vi "Configure.vi"(8 "error in (no error)":errorcluster, 9 "DAQ Parameters":T1={"Points Per A-Scan"=1024, "A-Scans Per B-Scan"=250, "Number of B-Scans"=1, "A-Scans Per Transfer"=1, "Trigger Voltage"=0.0, "Trigger Source"=enum."External", "Trigger Slope"=enum."Rising", "Channel"=enum."Channel 1", "Clock"=enum."Internal Clock", "Bits per Sample"=0.0, "Range"=0.0}, 10 "Scanning Parameters":T6={"Fast Axis Offset"=10.0, "Slow Axis Offset"=0.0, "Slow Axis Amp"=20.0, "Fast Axis Amp"=20.0, "Scan Pattern"=enum."Raster"} {"Fast Axis Amp" max=20 format="%#.2f"; "Slow Axis Amp" max=20 format="%#.2f"; "Slow Axis Offset" max=10 format="%#.2f"; "Fast Axis Offset" max=10 format="%#.2f"}, 11 "NI Galvo in":refnum<class "NI Galvo.lvclass">) -> (0 "error out":errorcluster, 3 "NI Galvo out":refnum<class "NI Galvo.lvclass">)   [LabVIEW 2014, in "NI Galvo.lvclass"]
uses:
  NI Galvo.lvclass
  Scanning Cluster.ctl
  DAQ/DAQ Parameters.ctl
  DAQ/Trigger Source.ctl
  DAQ/Trigger Slope.ctl
  Type Defs/OCT DAQ Channel Data Type.ctl
  DAQ/Clock Control.ctl
  Galvo.lvclass
  DAQ/DAQ Class.lvclass
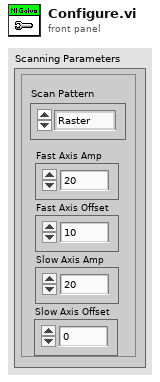
[diagram p1: front panel]
types:
  T1 = typedef "DAQ Class.lvclass/DAQ Parameters.ctl" = cluster{"Points Per A-Scan":u32, "A-Scans Per B-Scan":u32, "Number of B-Scans":u32, "A-Scans Per Transfer":u32, "Trigger Voltage":sgl, "Trigger Source":T2, "Trigger Slope":T3, "Channel":T4, "Clock":T5, "Bits per Sample":dbl, "Range":dbl}
  T2 = typedef "DAQ Class.lvclass/Trigger Source.ctl" = enum16{"External", "Channel A", "Channel B"}
  T3 = typedef "DAQ Class.lvclass/Trigger Slope.ctl" = enum16{"Rising", "Falling"}
  T4 = typedef "OCT DAQ Channel Data Type.ctl" = enum16{"Channel 1", "Channel 2", "Channel 1 and 2"}
  T5 = typedef "DAQ Class.lvclass/Clock Control.ctl" = enum16{"Internal Clock", "External Clock"}
  T6 = typedef "Galvo.lvclass/Scanning Cluster.ctl" = cluster{"Fast Axis Offset":sgl, "Slow Axis Offset":sgl, "Slow Axis Amp":sgl, "Fast Axis Amp":sgl, "Scan Pattern":enum16{"Raster"}}
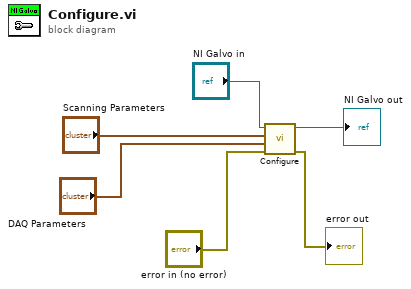
[diagram p0: block diagram]
diagram:
  n1 = call-parent "Configure.vi"("error in (no error)"="error in (no error)", "DAQ Parameters"="DAQ Parameters", "Scanning"="Scanning Parameters", "Galvo in"="NI Galvo in") -> ("error out"=→"error out":errorcluster, "Galvo out"=→"NI Galvo out":refnum<class "NI Galvo.lvclass">)  [unwired: 6 in]
